vi "LabVIEWArduino1SLIDER.vi"() -> ()   [LabVIEW 2020]
uses:
  <vilib>/Instr/_visa.llb/VISA Configure Serial Port (Instr).vi
panel:
  in  "Slide":u8(slide)
  in  "GO UP":bool
  in  "GO DOWN":bool
  in  "MAX SPEED":bool
  in  "SLOWEST SPEED":bool
  out "Waveform Graph":dbl[](graph)
  in  "VISA resource name":refnum<visa-resource-name>="COM3"
  in  "data bits (8)":u16=8 min=5 max=8 step=1
  in  "stop bits (10: 1 bit)":u16(ring)=10 items=["1.0"=10, "1.5"=15, "2.0"=20]
  in  "flow control (0:none)":u16(ring) items=["None", "XON/XOFF", "RTS/CTS", "XON/XOFF & RTS/CTS", "DTR/DSR", "XON/XOFF & DTR/DSR"]
  in  "parity (0:none)":enum16{"None", "Odd", "Even", "Mark", "Space"}(ring)
  out "TempArray":dbl[](array[numeric]) caption="Temperature Array"
  out "CurTemp":dbl caption="Current Temperature\n(Celsius)"
  out "concatenated string":string
  in  "stop":bool
  in  "LabVIEW Stop":bool
  in  "Emergency Stop!":bool
  in  "Decellerate":bool
  in  "Motor Control Duino":refnum<visa-resource-name>
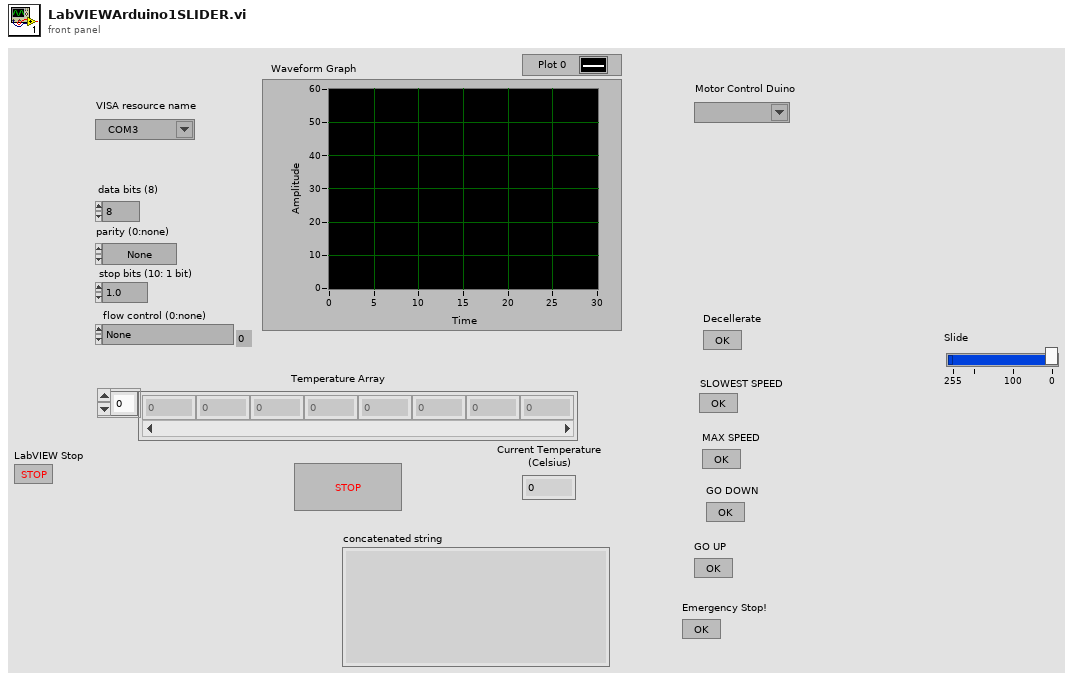
[diagram p1: front panel]
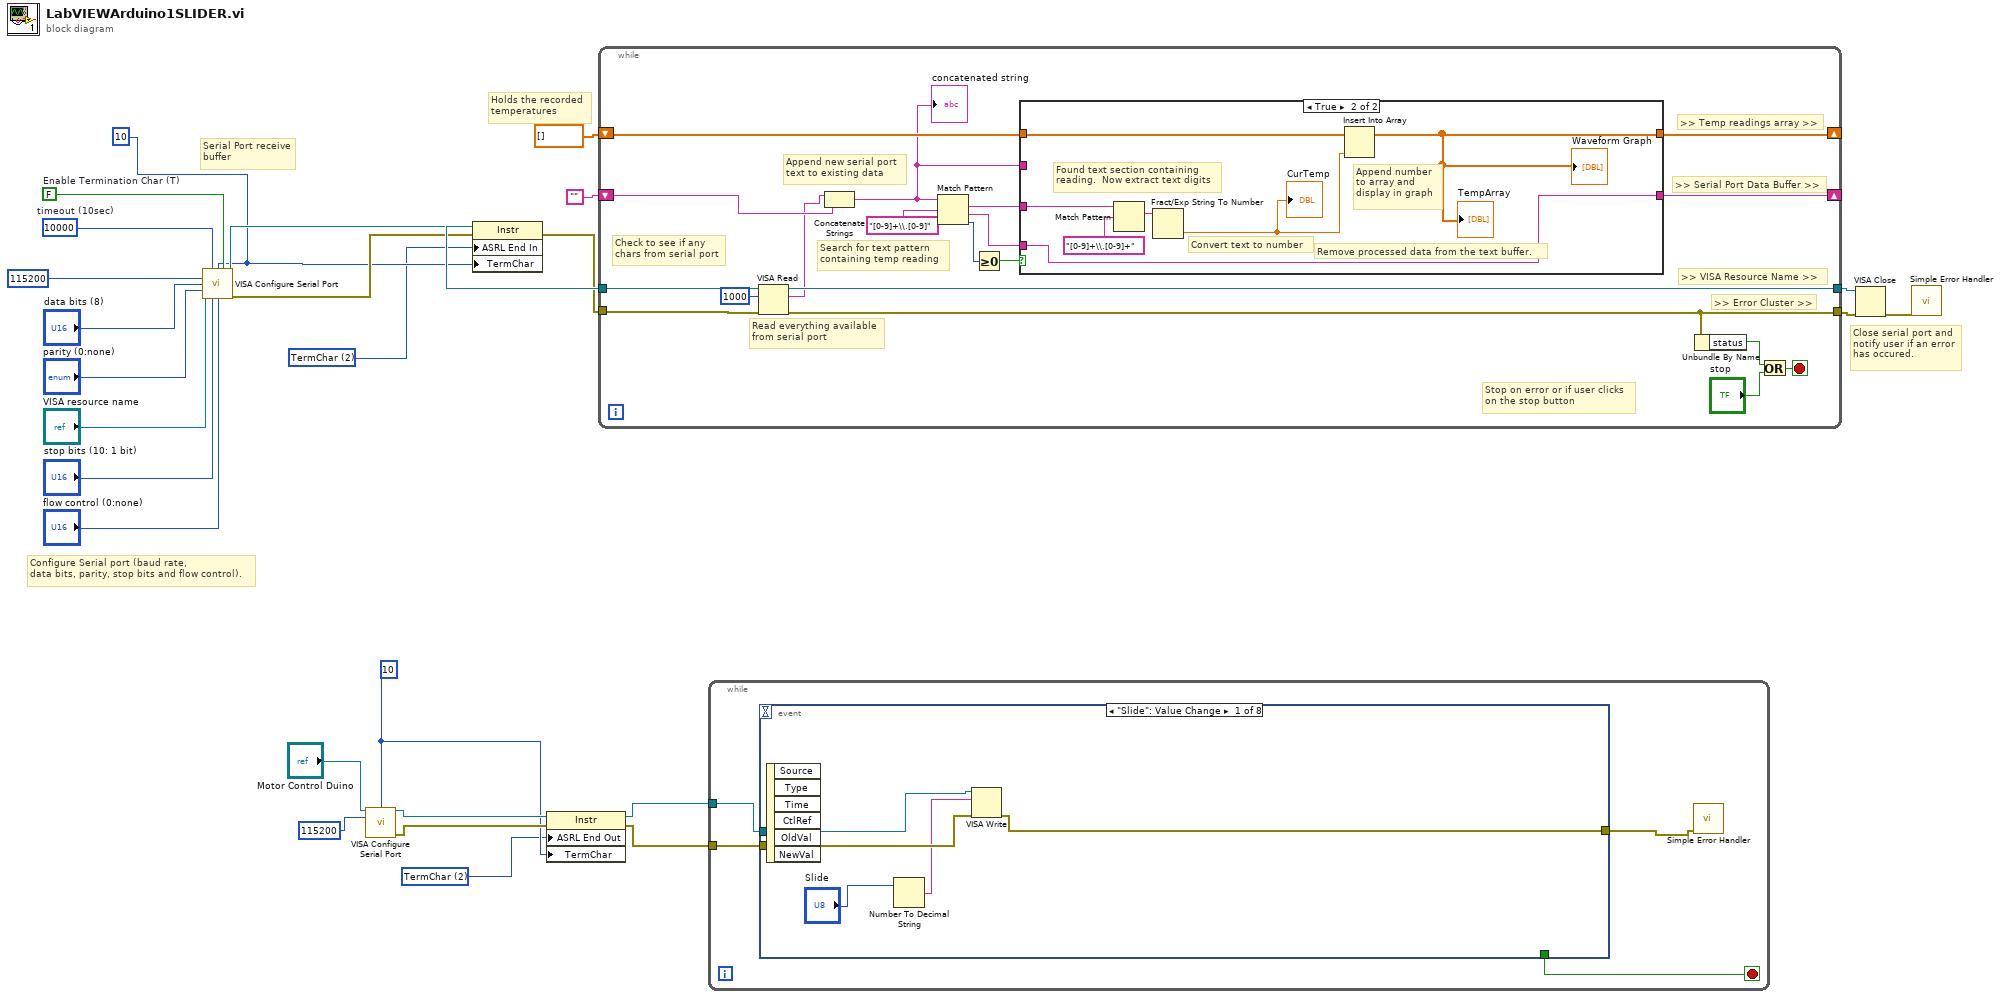
[diagram p0: block diagram]
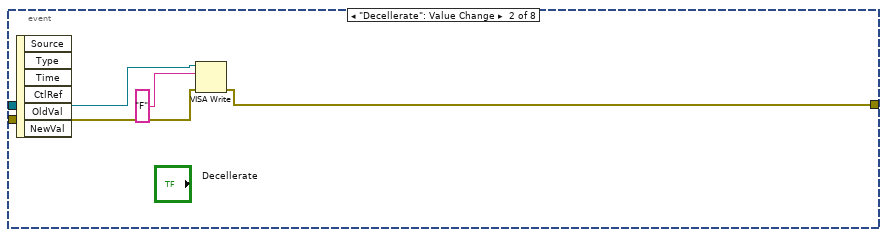
[diagram p3: hidden frame]
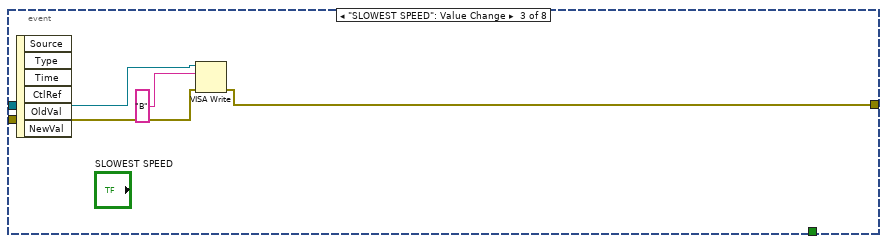
[diagram p4: hidden frame]
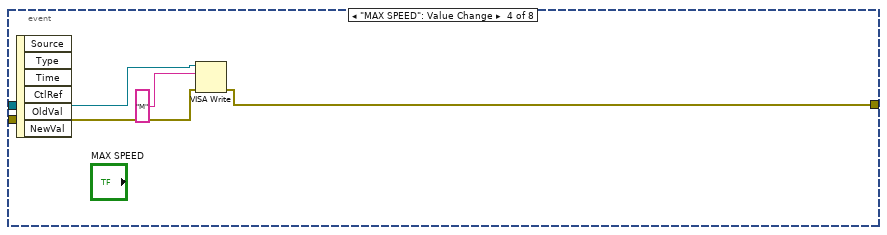
[diagram p5: hidden frame]
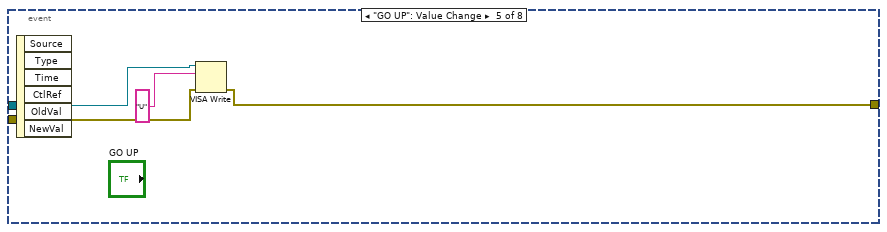
[diagram p6: hidden frame]
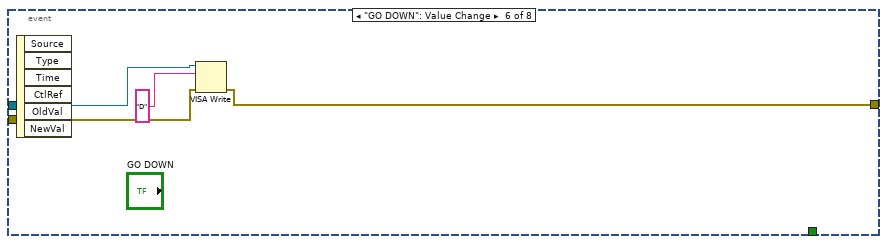
[diagram p7: hidden frame]
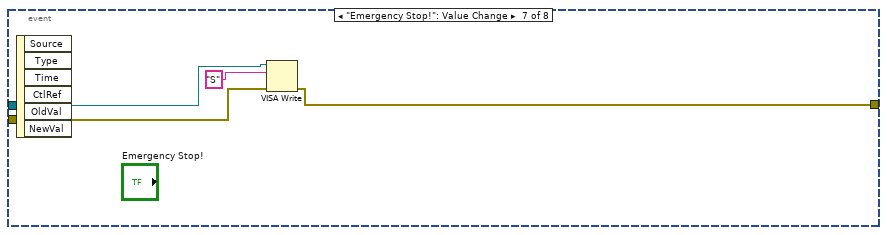
[diagram p8: hidden frame]
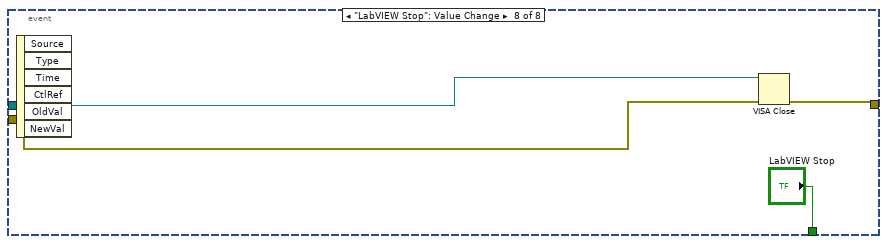
[diagram p9: hidden frame]
diagram:
  w1 = u16 2 items=["None", "Last Bit", "TermChar", "Break"] ("Serial Settings:End Mode for Writes")
  w2 = u8 10 ("termination char\n(0xA = '\\n' = LF)")
  w7 = u16 2 items=["None", "Last Bit", "TermChar"] ("Serial Settings:End Mode for Reads")
  w8 = u8 10 ("Message Based Settings:Termination Character")
  w21 = FALSE  # Enable Termination Char (T)
  w22 = u32 10000  # timeout (10sec)
  # "Close serial port and\nnotify user if an error\nhas occured."
  # "Serial Port receive\nbuffer"
  # "Holds the recorded\ntemperatures"
  # "Configure Serial port (baud rate,\ndata bits, parity, stop bits and flow control)."
  n1 = call-poly "VISA Configure Serial Port"("VISA resource name"="VISA resource name", "timeout (10sec)"=w22, "termination char\n(0xA = '\\n' = LF)"=w8, "Enable Termination\nChar (T)"=w21, "baud rate (9600)"=u32 115200, "data bits (8)"="data bits (8)", "parity (0:none)"="parity (0:none)", "stop bits (10: 1 bit)"="stop bits (10: 1 bit)", "flow control (0:none)"="flow control (0:none)") -> ("VISA resource name out"=w10:refnum<visa-resource-name>, "error out"=w9:errorcluster)  [unwired: 5 in]
  n2 = call-poly "VISA Configure Serial Port"("VISA resource name"="Motor Control Duino", "termination char\n(0xA = '\\n' = LF)"=w2, "baud rate (9600)"=u32 115200) -> ("VISA resource name out"=w6:refnum<visa-resource-name>, "error out"=w5:errorcluster)  [unwired: 11 in]
  n3 = property class="Instr"(reference=w10, error in=w9, "ASRL End In"=w7, "TermChar"=w8) -> (reference out=w12:refnum<visa-resource-name>, error out=w11:errorcluster)
  n4 = property class="Instr"(reference=w6, error in=w5, "ASRL End Out"=w1, "TermChar"=w2) -> (reference out=w4:refnum<visa-resource-name>, error out=w3:errorcluster)
  n5 = while {
    tunnel: [w43] -> w25
    tunnel: [w46] -> w24
    shift-right: [w37] -> _
    shift-left: "" -> [w44]
    tunnel: w12 -> [w45]
    tunnel: w11 -> [w36]
    shift-right: [w39] -> _
    shift-left: dbl[] [] -> [w38]
    stop <- w42 stop-if-true
    # "Search for text pattern\ncontaining temp reading"
    # "Append new serial port\ntext to existing data"
    # "Read everything available\nfrom serial port"
    # "Stop on error or if user clicks \non the stop button"
    # ">> Error Cluster >>"
    # ">> VISA Resource Name >>"
    # ">> Temp readings array >>"
    # ">> Serial Port Data Buffer >>"
    # "Check to see if any\nchars from serial port"
    n6 = VISA Read(VISA resource name=w45, byte count=u32 1000, error in (no error)=w36) -> (VISA resource name out=w46:refnum<visa-resource-name>, read buffer=w29:string, error out=w43:errorcluster)  [unwired: 1 out]
    n7 = Concatenate Strings(w29, w44) -> (w30:string)
    "concatenated string" <- w30
    n8 = Match Pattern(string=w30, regular expression="[0-9]+\\.[0-9]") -> (match substring=w32:string, after substring=w31:string, offset past match=w34:i32)  [unwired: 1 in, 1 out]
    n9 = Greater Or Equal To 0?(x=w34) -> (x >= 0?=w33:bool)
    n10 = case shown="True" w33 {
      tunnel: w32 -> [_ w54]
      tunnel: w31 -> [_ w55]
      tunnel: w30 -> [w48 _]
      tunnel: [w48 w55] -> w37
      tunnel: [w47 w49] -> w39
      tunnel: w38 -> [w47 w52]
      frame False {
        # "Did not find text pattern in the buffer.  Try again in the next loop after new data \nhas been received."
      }
      frame True {
        # "Remove processed data from the text buffer."
        # "Append number\nto array and\ndisplay in graph"
        # "Convert text to number"
        # "Found text section containing \nreading.  Now extract text digits"
        n11 = Match Pattern(string=w54, regular expression="[0-9]+\\.[0-9]+") -> (match substring=w53:string)  [unwired: 1 in, 3 out]
        n12 = Fract/Exp String To Number(string=w53) -> (number=w50:dbl)  [unwired: 3 in, 1 out]
        "CurTemp" <- w50
        n13 = Insert Into Array(array=w52, new element=w50) -> (w49:dbl[])  [unwired: 1 in]
        "TempArray" <- w49
        "Waveform Graph" <- w49
      }
    }
    n14 = Unbundle By Name(w43) -> ("status"=w41:bool)
    n15 = Or(x=w41, y="stop") -> (x .or. y?=w42:bool)
  }
  n16 = while {
    tunnel: w4 -> [w59]
    tunnel: w3 -> [w58]
    stop <- w56 stop-if-true
    n17 = event shown="[0] \"Slide\": Value Change" {
      selector: _ -> [_ _ _ _ _ _ _ _]
      dyn-events: _ -> [_ _ _ _ _ _ _ _]
      timeout: _ -> [_ _ _ _ _ _ _ _]
      tunnel: [w64 w68 w72 w76 w80 w84 w88 w92] -> w57
      tunnel: w59 -> [w63 w66 w70 w74 w78 w82 w86 w91]
      tunnel: w58 -> [w62 w65 w69 w73 w77 w81 w85 w90]
      tunnel: [_ _ _ _ _ _ _ "LabVIEW Stop"] -> w56
      event "Slide": Value Change {
        n18 = event-data() -> ()  [unwired: 1 in, 6 out]
        n19 = Number To Decimal String(number="Slide") -> (decimal integer string=w60:string)  [unwired: 1 in]
        n20 = VISA Write(VISA resource name=w63, write buffer=w60, error in (no error)=w62) -> (error out=w64:errorcluster)  [unwired: 2 out]
      }
      event "Decellerate": Value Change {
        n21 = event-data() -> ()  [unwired: 1 in, 6 out]
        n22 = VISA Write(VISA resource name=w66, write buffer="F", error in (no error)=w65) -> (error out=w68:errorcluster)  [unwired: 2 out]
      }
      event "SLOWEST SPEED": Value Change {
        n23 = event-data() -> ()  [unwired: 1 in, 6 out]
        n24 = VISA Write(VISA resource name=w70, write buffer="B", error in (no error)=w69) -> (error out=w72:errorcluster)  [unwired: 2 out]
      }
      event "MAX SPEED": Value Change {
        n25 = event-data() -> ()  [unwired: 1 in, 6 out]
        n26 = VISA Write(VISA resource name=w74, write buffer="M", error in (no error)=w73) -> (error out=w76:errorcluster)  [unwired: 2 out]
      }
      event "GO UP": Value Change {
        n27 = event-data() -> ()  [unwired: 1 in, 6 out]
        n28 = VISA Write(VISA resource name=w78, write buffer="U", error in (no error)=w77) -> (error out=w80:errorcluster)  [unwired: 2 out]
      }
      event "GO DOWN": Value Change {
        n29 = event-data() -> ()  [unwired: 1 in, 6 out]
        n30 = VISA Write(VISA resource name=w82, write buffer="D", error in (no error)=w81) -> (error out=w84:errorcluster)  [unwired: 2 out]
      }
      event "Emergency Stop!": Value Change {
        n31 = event-data() -> ()  [unwired: 1 in, 6 out]
        n32 = VISA Write(VISA resource name=w86, write buffer="S", error in (no error)=w85) -> (error out=w88:errorcluster)  [unwired: 2 out]
      }
      event "LabVIEW Stop": Value Change {
        n33 = event-data() -> ()  [unwired: 1 in, 6 out]
        n34 = VISA Close(VISA resource name=w91, error in (no error)=w90) -> (error out=w92:errorcluster)
      }
    }
    n35 = call <vilib>:"Simple Error Handler.vi"("error in (no error)"=w57) -> ()  [unwired: 4 in, 5 out]
  }
  n36 = VISA Close(VISA resource name=w24, error in (no error)=w25) -> (error out=w23:errorcluster)
  n37 = call <vilib>:"Simple Error Handler.vi"("error in (no error)"=w23) -> ()  [unwired: 4 in, 5 out]
